vi "Left Main Sequence.vi"   [LabVIEW 2015]
uses:
  <vilib>/FPGAPlugInAG/myRIO-1900/niLvFpga_Open_myRIO-1900.vi
  <vilib>/rvi/interface/common/dynamic/niFpgaDynamicAddResources.vi
  <vilib>/myRIO/Common/Instrument Driver Framework/Utilities/vis/FPGA Ref Manager.vi
  <vilib>/Utility/error.llb/Error Cluster From Error Code.vi
  <vilib>/myRIO/Common/Instrument Driver Framework/Utilities/vis/Ref Counter.vi
  <vilib>/rvi/interface/nirviOpenFPGA/nirviOpenFPGA.xnode
  LidarLitev3test_FPGATarget_FPGAMainwLidarLi_c8ybSBS-918.lvbitx
  <vilib>/myRIO/Instrument Drivers/Utilities/Utilities.lvlib
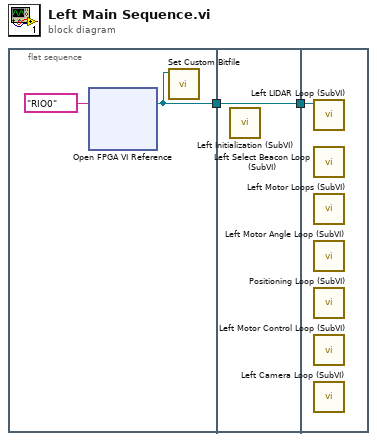
[diagram p0: block diagram]
diagram:
  n1 = flat-sequence {
    tunnel: [w4] -> w2
    tunnel: w2 -> [w5]
    tunnel: [w5] -> w1
    tunnel: w1 -> [w6]
    frame #0 {
      n2 = xnode "Open FPGA VI Reference"("resource name"=tag "RIO0") -> ("FPGA VI Reference Out"=w4:refnum<k20>)  [unwired: 1 in, 1 out]
      n3 = call <vilib>:"Set Custom Bitfile.vi"("Custom FPGA Reference In"=w4) -> ()  [unwired: 9 in, 2 out]
    }
    frame #1 {
      n4 = call "Left Initialization (SubVI).vi"() -> ()  [unwired: 12 in]
    }
    frame #2 {
      n5 = call "Left LIDAR Loop (SubVI).vi"("Refnum in"=w6) -> ()  [unwired: 11 in]
      n6 = call "Left Select Beacon Loop (SubVI).vi"() -> ()  [unwired: 12 in]
      n7 = call "Left Motor Loops (SubVI).vi"() -> ()  [unwired: 12 in]
      n8 = call "Left Motor Angle Loop (SubVI).vi"() -> ()  [unwired: 12 in]
      n9 = call "Positioning Loop (SubVI).vi"() -> ()  [unwired: 12 in]
      n10 = call "Left Motor Control Loop (SubVI).vi"() -> ()  [unwired: 12 in]
      n11 = call "Left Camera Loop (SubVI).vi"() -> ()  [unwired: 12 in]
    }
  }
